vi "DP-Find Thresholds.vi"(8 "Criteria":dbl[](array[numeric]), 9 "L2":dbl[](array[numeric]), 10 "DP":dbl[](array[numeric]), 11 "Noise criterion":dbl) -> (0 "Thresholds":dbl[](array[numeric]))   [LabVIEW 2020]
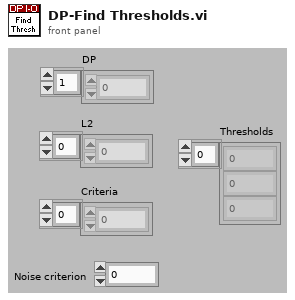
[diagram p1: front panel]
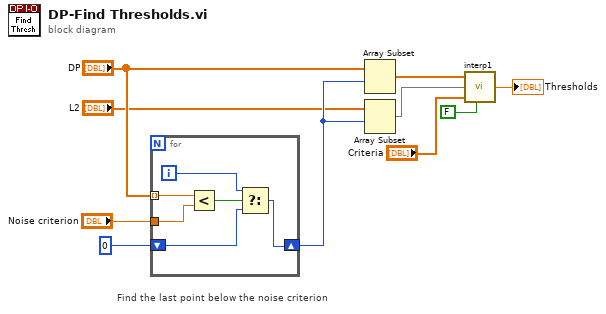
[diagram p0: block diagram]
diagram:
  # "Find the last point below the noise criterion"
  n1 = for {
    tunnel: "DP" -> [w16] mode=indexing
    tunnel: "Noise criterion" -> [w15]
    shift-right: [w11] -> w7
    shift-left: 0 -> [w12]
    i -> [w13]
    n2 = Less?(x=w16, y=w15) -> (x < y?=w14:bool)
    n3 = Select(t=w13, s=w14, f=w12) -> (s? t:f=w11:i32)
  }
  n4 = Array Subset(array="DP", index=w7) -> (w5:dbl[])  [unwired: 1 in]
  n5 = Array Subset(array="L2", index=w7) -> (w2:dbl[])  [unwired: 1 in]
  n6 = call "interp1.vi"("X"=w5, "Y"=w2, "U"="Criteria", "extrapolate"=FALSE) -> ("V"=→"Thresholds":dbl)  [unwired: 1 in]
